vi "Part 6 Matrix Size.vi"() -> ()   [LabVIEW 2020]
uses:
  <vilib>/Analysis/Matrix/Datatypes/RealMatrix.ctl
  <vilib>/Analysis/Matrix/NI_Matrix.lvlib
panel:
  out "number of columns":i32
  out "number of rows":i32
  in  "matrix":T1
  # "Matrix Size"
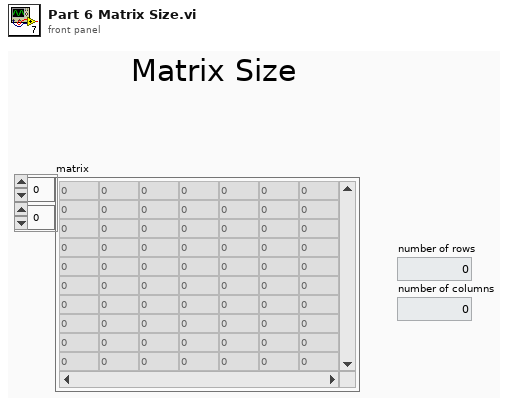
[diagram p1: front panel]
types:
  T1 = typedef "NI_Matrix.lvlib/RealMatrix.ctl" = dbl[][]
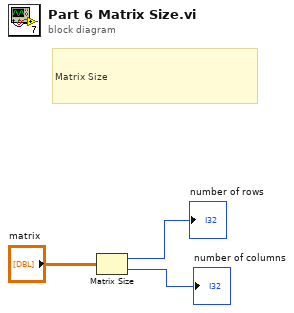
[diagram p0: block diagram]
diagram:
  # "Matrix Size"
  n1 = Matrix Size(0:"matrix") -> (1:→"number of rows":i32, 2:→"number of columns":i32)
